vi "Recompose Item.vi"(8 "error in (no error)":errorcluster, 9 "Nesting Level":i32, 10 "All Data":refnum<class "Data Item.lvclass">[](array[class]), 11 "Data Item in":refnum<class "Data Item.lvclass">) -> (0 "error out":errorcluster, 1 "XML String":string, 2 "All Data out":refnum<class "Data Item.lvclass">[](array[class]), 3 "Data Item out":refnum<class "Data Item.lvclass">)   [LabVIEW 2026, in "VILab.lvlib" / "Data Item.lvclass"]
uses:
  Data Item.lvclass
  VILab.lvlib
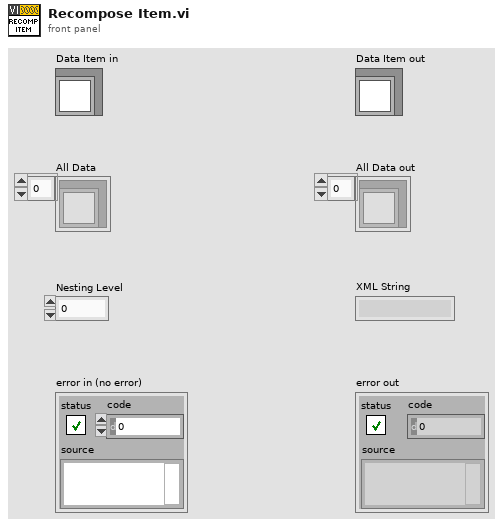
[diagram p1: front panel]
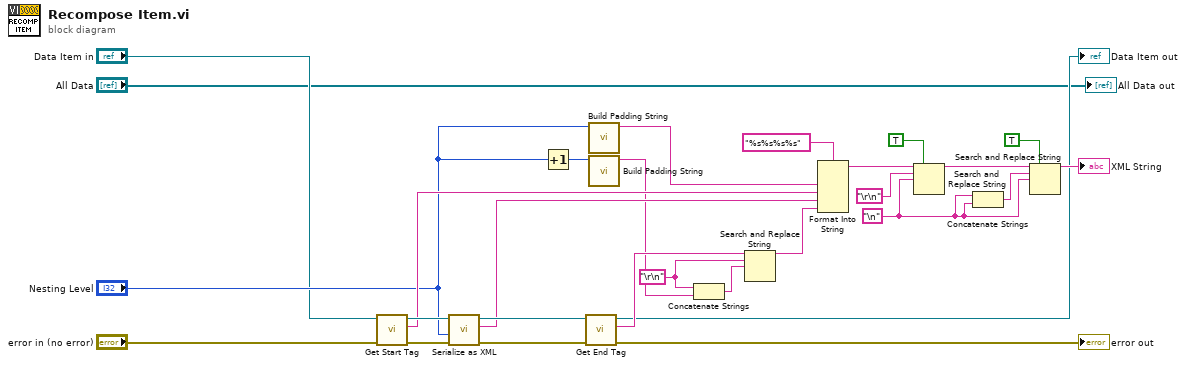
[diagram p0: block diagram]
diagram:
  w9 = "\n"
  w20 = "\r\n"
  n1 = call-dynamic "Get Start Tag.vi"("error in (no error)"="error in (no error)", "Data Item in"="Data Item in") -> ("error out"=w26:errorcluster, "Start Tag"=w23:string, "Data Item out"=w25:refnum<class "Data Item.lvclass">)  [unwired: 7 in]
  n2 = call-dynamic "Serialize as XML.vi"("error in (no error)"=w26, "Nesting Level"="Nesting Level", "Data Item in"=w25) -> ("error out"=w28:errorcluster, "XML Fragment"=w22:string, "Data Item out"=w27:refnum<class "Data Item.lvclass">)  [unwired: 6 in]
  n3 = Increment(x="Nesting Level") -> (x+1=w16:i32)
  n4 = call-dynamic "Get End Tag.vi"("error in (no error)"=w28, "Data Item in"=w27) -> ("error out"=→"error out":errorcluster, "End Tag"=w21:string, "Data Item out"=→"Data Item out":refnum<class "Data Item.lvclass">)  [unwired: 7 in]
  n5 = call "Build Padding String.vi"("Nesting Level"="Nesting Level") -> ("Padding"=w17:string)  [unwired: 10 in]
  n6 = call "Build Padding String.vi"("Nesting Level"=w16) -> ("Padding"=w15:string)  [unwired: 10 in]
  n7 = Concatenate Strings(w20, w15) -> (w19:string)
  n8 = Search and Replace String(input string=w21, search string=w20, replace string=w19) -> (result string=w18:string)  [unwired: 5 in, 3 out]
  n9 = Format Into String(format string="%s%s%s%s", w17, w23, w22, w18) -> (resulting string=w14:string)  [unwired: 2 in, 1 out]
  n10 = Search and Replace String(replace all?=TRUE ("replace all? (F)"), input string=w14, search string="\r\n", replace string=w9) -> (result string=w10:string)  [unwired: 4 in, 3 out]
  n11 = Concatenate Strings(w9, w9) -> (w8:string)
  n12 = Search and Replace String(replace all?=TRUE ("replace all? (F)"), input string=w10, search string=w8, replace string=w9) -> (result string=→"XML String":string)  [unwired: 4 in, 3 out]
  "All Data out" <- "All Data"
